vi "2d_ref_model.vi"(3 "error in (no error)":errorcluster, 4 "f_band":dbl, 5 "dt":dbl, 6 "x":dbl format="%0.2f") -> (0 "error out":errorcluster, 2 "Filtered x":dbl format="%0.2f")   [LabVIEW 2019]
uses:
  <vilib>/ptbypt/NI_PtbyPt.lvlib
panel:
  out "a2":dbl
  out "a1":dbl
  out "a0":dbl
  out "b1":dbl
  out "b2":dbl
  out "b0":dbl
  out "wn":dbl
  out "T":dbl
  out "zeta":dbl
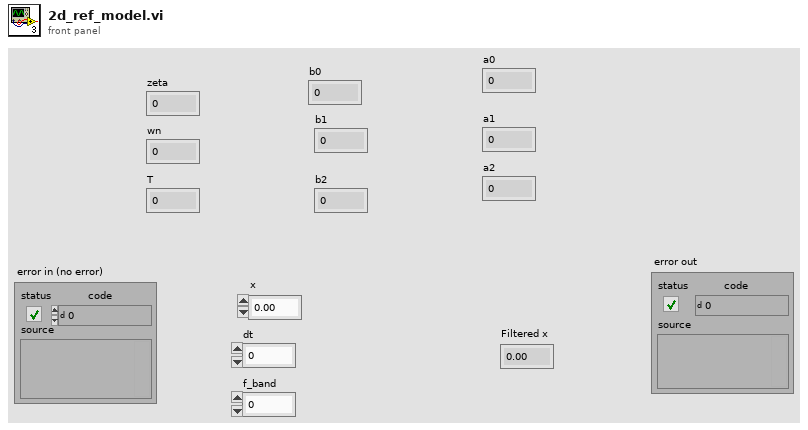
[diagram p1: front panel]
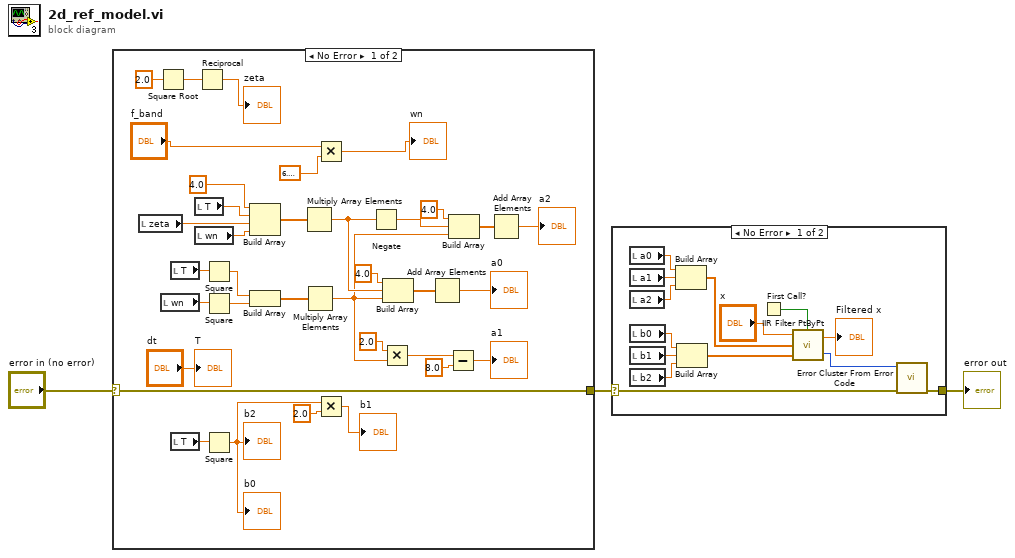
[diagram p0: block diagram]
diagram:
  n1 = case shown="No Error" "error in (no error)" {
    selector: "error in (no error)" -> [w7 w39]
    tunnel: [w7 w39] -> w2
    frame No Error {
      n2 = local read "zeta"() -> (w28:dbl)
      n3 = Square Root(x=2.0) -> (sqrt(x)=w38:dbl)
      n4 = local read "wn"() -> (w21:dbl)
      n5 = local read "T"() -> (w24:dbl)
      n6 = local read "T"() -> (w34:dbl)
      n7 = local read "T"() -> (w29:dbl)
      n8 = local read "wn"() -> (w27:dbl)
      n9 = Reciprocal(x=w38) -> (1/x=→"zeta":dbl)
      n10 = Square(x=w24) -> (x^2=w23:dbl)
      n11 = Square(x=w21) -> (x^2=w22:dbl)
      n12 = Square(x=w34) -> (x^2=w31:dbl)
      "b0" <- w31
      "b2" <- w31
      n13 = Build Array(4.0 ("element"), w29, w28, w27) -> (w26:dbl[])
      n14 = Build Array(w23, w22) -> (w25:dbl[])
      n15 = Multiply Array Elements(1:w26) -> (0:w10:dbl)
      n16 = Multiply Array Elements(1:w25) -> (0:w9:dbl)
      n17 = Multiply(x="f_band", y=6.283185307179586) -> (x*y=→"wn":dbl)
      n18 = Multiply(x=w31, y=2.0) -> (x*y=→"b1":dbl)
      n19 = Negate(x=w10) -> (-x=w11:dbl)
      n20 = Multiply(x=2.0, y=w9) -> (x*y=w16:dbl)
      n21 = Build Array(4.0 ("element"), w10, w9) -> (w19:dbl[])
      n22 = Add Array Elements(numeric array=w19) -> (sum=→"a0":dbl)
      n23 = Subtract(x=w16, y=8.0) -> (x-y=→"a1":dbl)
      n24 = Build Array(4.0 ("element"), w11, w9) -> (w13:dbl[])
      n25 = Add Array Elements(numeric array=w13) -> (sum=→"a2":dbl)
      "T" <- "dt"
    }
    frame Error {
    }
  }
  n26 = case shown="No Error" w2 {
    selector: w2 -> [w42 w54]
    tunnel: [w40 w54] -> w1
    frame No Error {
      n27 = local read "a0"() -> (w48:dbl)
      n28 = local read "a1"() -> (w47:dbl)
      n29 = local read "a2"() -> (w46:dbl)
      n30 = local read "b0"() -> (w45:dbl)
      n31 = local read "b1"() -> (w44:dbl)
      n32 = local read "b2"() -> (w43:dbl)
      n33 = Build Array(w48, w47, w46) -> (w50:dbl[])
      n34 = Build Array(w45, w44, w43) -> (w49:dbl[])
      n35 = First Call?() -> (First Call?: T/F=w53:bool)
      n36 = call <vilib>:"IIR Filter PtByPt.vi"("initialize"=w53, "Forward Coefficients"=w49, "Reverse Coefficients"=w50, "x"="x") -> ("error"=w41:i32, "Filtered x"=→"Filtered x":dbl)
      n37 = call <vilib>:"Error Cluster From Error Code.vi"("error in (no error)"=w42, "error code (0)"=w41) -> ("error out"=w40:errorcluster)  [unwired: 7 in]
    }
    frame Error {
    }
  }
  "error out" <- w1
